vi "_PC_RTLoop_ReadVacuumSys.vi"(0 "string for turbo pump status":refnum<vi>, 1 "XYGraph for pressure":refnum<vi>[](array[refnum]), 2 "String refin":refnum<vi>, 3 "Function":enum16{"Init", "Get Data", "Close"}(ring), 5 "XYGraph for Turbo power":refnum<vi>, 9 "XYGraph for Turbo speed":refnum<vi>, 11 "error in (no error)":errorcluster) -> (15 "error out":errorcluster)   [LabVIEW 2018]
uses:
  <resource>/objmgr/ni.var.rc
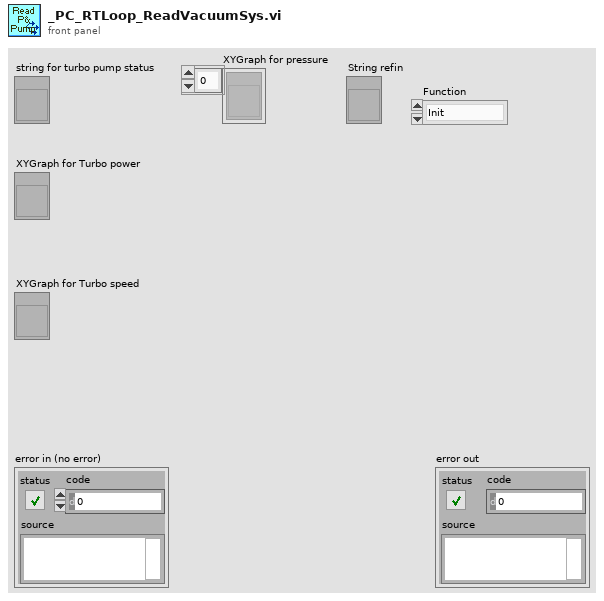
[diagram p1: front panel]
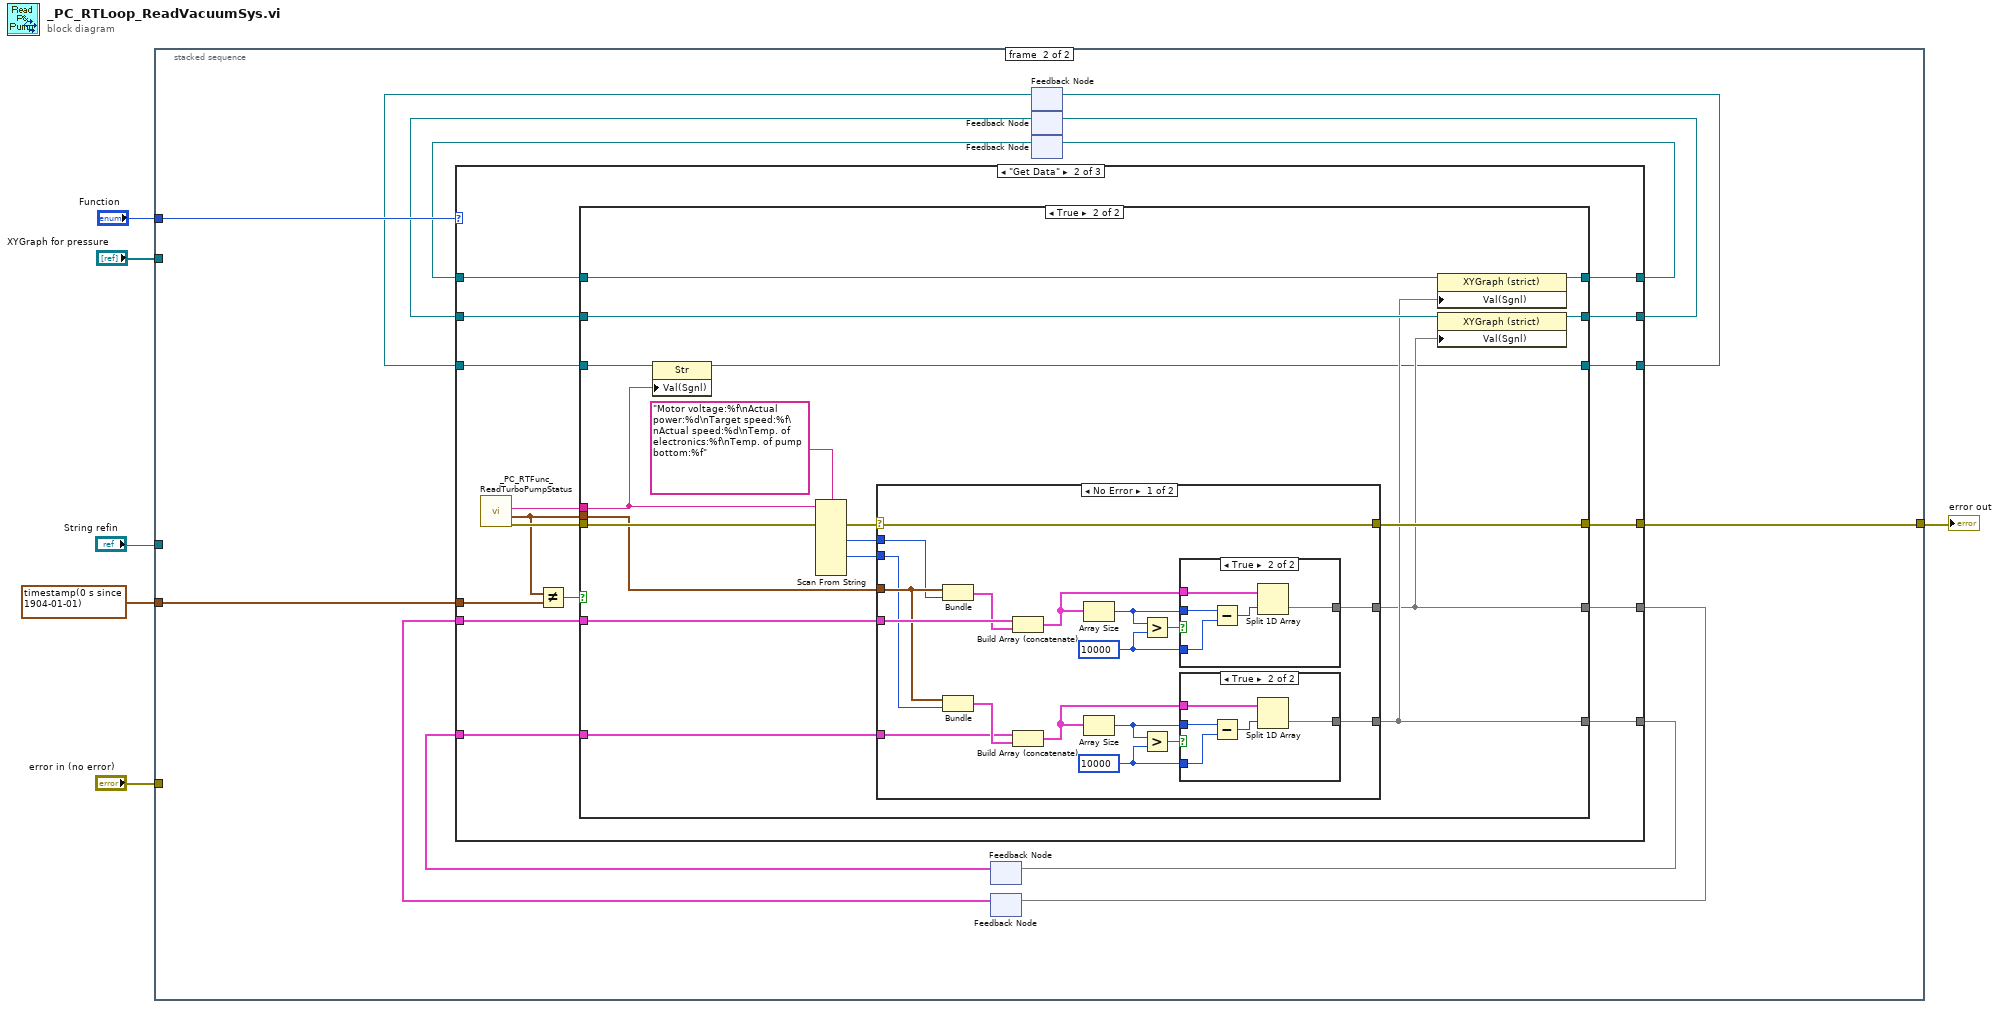
[diagram p0: block diagram]
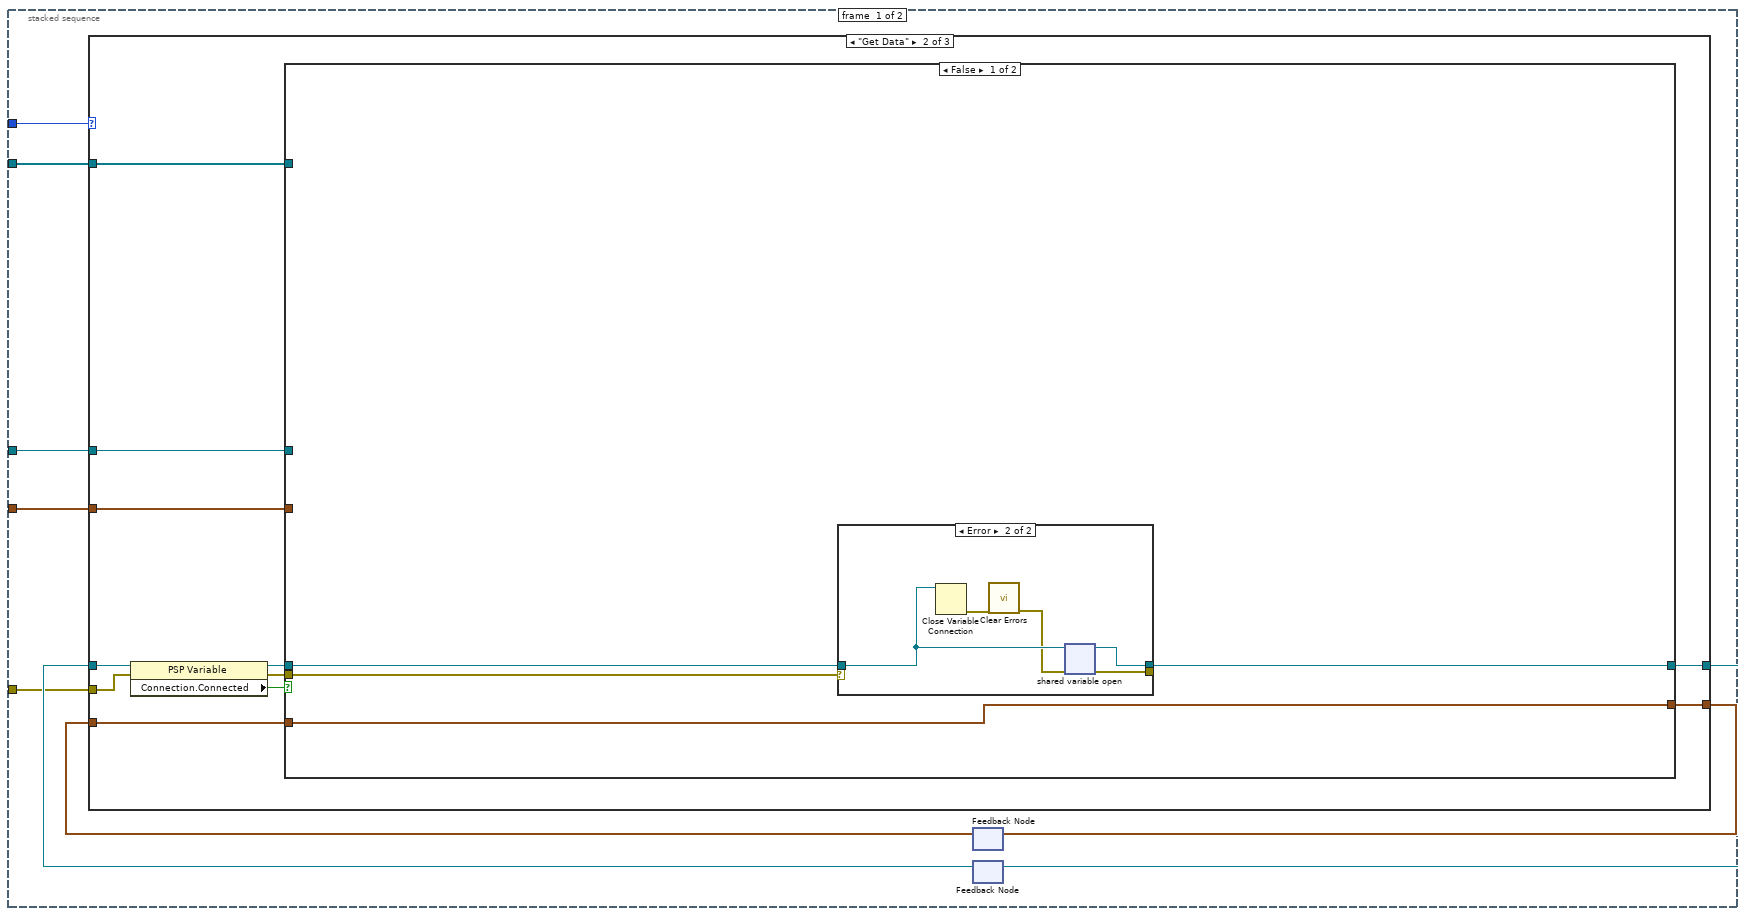
[diagram p2: hidden frame]
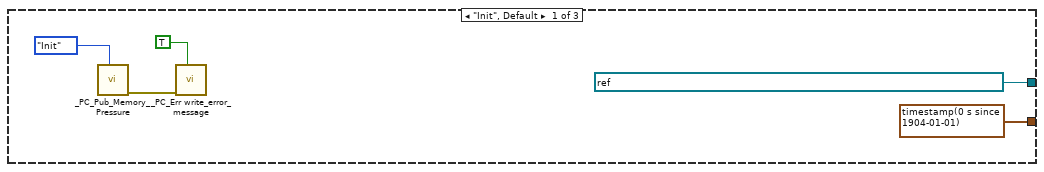
[diagram p3: hidden frame]
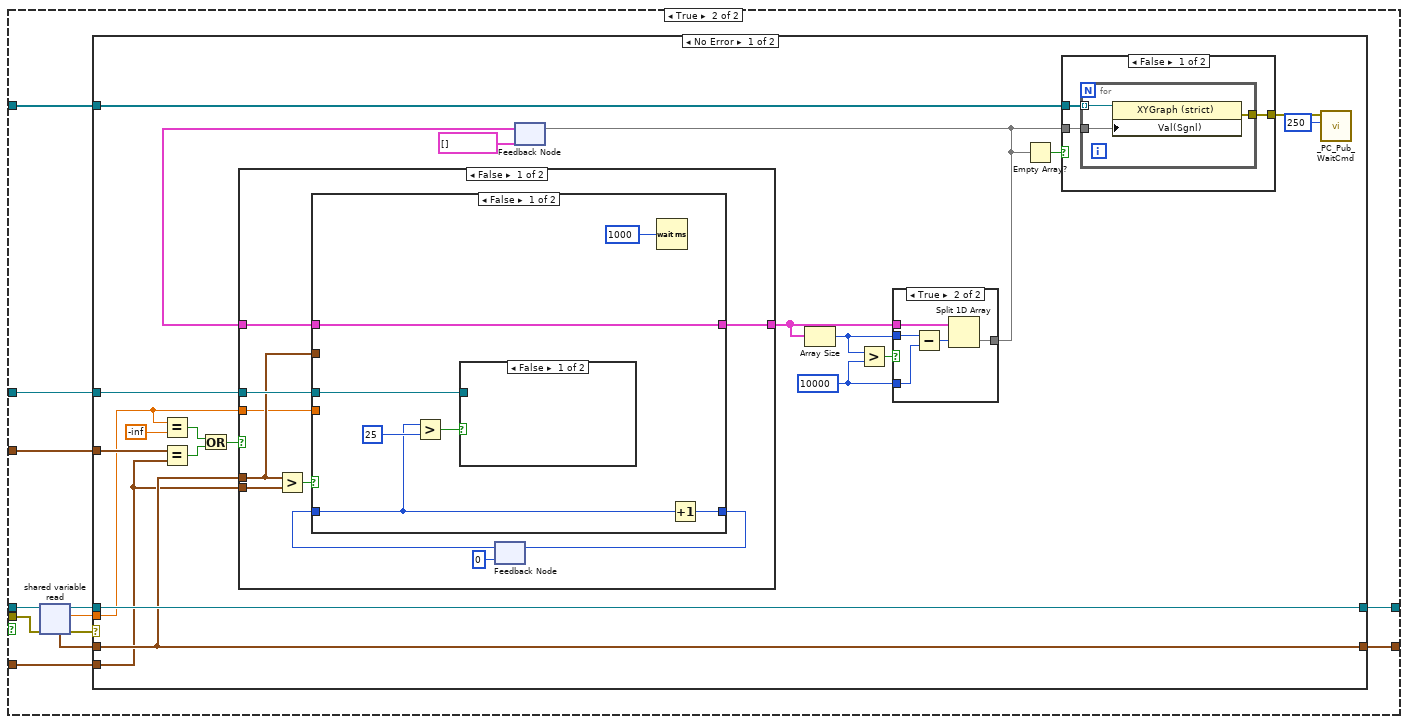
[diagram p5: hidden frame]
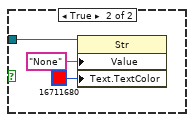
[diagram p8: hidden frame]
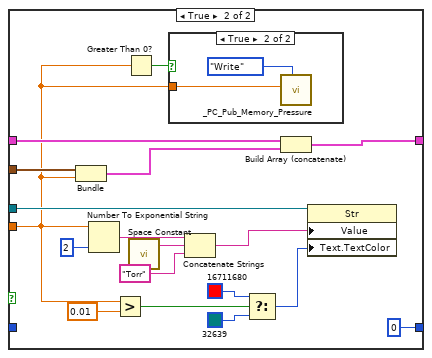
[diagram p9: hidden frame]
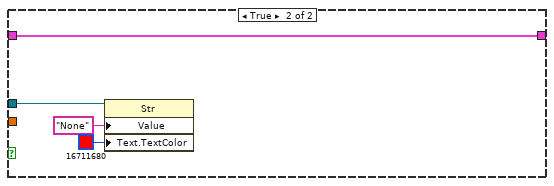
[diagram p11: hidden frame]
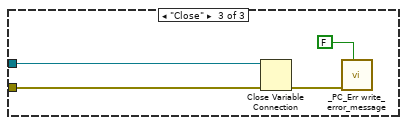
[diagram p13: hidden frame]
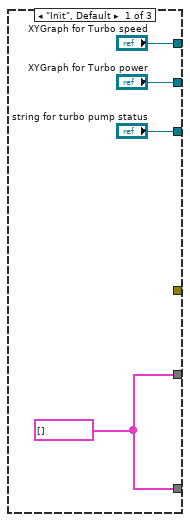
[diagram p14: hidden frame]
diagram:
  n1 = stacked-sequence {
    tunnel: "error in (no error)" -> [w13 _]
    tunnel: "Function" -> [w12 w149]
    tunnel: timestamp(0 s since 1904-01-01) -> [w9 w148]
    tunnel: "String refin" -> [w8 _]
    tunnel: "XYGraph for pressure" -> [w7 _]
    tunnel: [_ w143] -> w2
    frame #0 {
      n2 = feedback #1() -> (w10:timestamp)  [unwired: 1 in]
      n3 = feedback #2() -> (w14:refnum<k21>)  [unwired: 1 in]
      n4 = case shown="\"Get Data\"" w12 {
        tunnel: [refnum<k21> "ni.var.psp://NI-sbRIO/_RT_CtrlLoop_Pressure_Variables/Pressure_dbl" ("shared variable refnum in") w31 _] -> w15
        tunnel: w14 -> [_ w25 w136]
        tunnel: w13 -> [_ w23 w135]
        tunnel: [timestamp(0 s since 1904-01-01) w29 _] -> w11
        tunnel: w10 -> [_ w30 _]
        tunnel: w9 -> [_ w28 _]
        tunnel: w8 -> [_ w27 _]
        tunnel: w7 -> [_ w26 _]
        frame "Init", Default {
          n5 = call "_PC_Pub_Memory_Pressure.vi"("Function"=enum16{"Init", "Write", "Read"}."Init") -> ("error out"=w18:errorcluster)  [unwired: 9 in, 1 out]
          n6 = call "_PC_Err write_error_message.vi"("show msg( T )"=TRUE, "error in"=w18) -> ()  [unwired: 9 in, 1 out]
        }
        frame "Get Data" {
          n7 = property class="PSP Variable"(reference=w25, error in=w23) -> (reference out=w24:refnum<k21>, error out=w22:errorcluster, "Connection.Connected"=w21:bool)
          n8 = case shown="False" w21 {
            tunnel: [w32 w50] -> w31
            tunnel: w30 -> [w35 w48]
            tunnel: [w35 w47] -> w29
            tunnel: w28 -> [_ w46]
            tunnel: w27 -> [_ w45]
            tunnel: w26 -> [_ w44]
            tunnel: w24 -> [w33 w43]
            tunnel: w22 -> [w34 w42]
            frame False {
              n9 = case shown="Error" w34 {
                tunnel: w33 -> [w36 w40]
                tunnel: [w36 w38] -> w32
                tunnel: [_ w37] -> _
                frame No Error {
                }
                frame Error {
                  n10 = Close Variable Connection(11:w40) -> (0:w41:errorcluster)  [unwired: 1 in]
                  n11 = call <vilib>:"Clear Errors.vi"("error in (no error)"=w41) -> ("error out"=w39:errorcluster)  [unwired: 5 in, 1 out]
                  n12 = shared-variable-open(w40, w39) -> (w38:refnum<k21>, w37:errorcluster)
                }
              }
            }
            frame True {
              n13 = shared-variable-read(w43, w42) -> (w51:refnum<k21>, w52:errorcluster, w53:dbl, w49:timestamp)
              n14 = case shown="No Error" w52 {
                tunnel: w53 -> [w57 _]
                tunnel: w51 -> [w74 w131]
                tunnel: [w74 w131] -> w50
                tunnel: w49 -> [w72 w132]
                tunnel: w48 -> [w59 _]
                tunnel: [w72 w132] -> w47
                tunnel: w46 -> [w73 _]
                tunnel: w45 -> [w71 _]
                tunnel: w44 -> [w66 _]
                frame No Error {
                  w69 = 10000 ("y")
                  n15 = Equal?(x=w57, y=-inf) -> (x = y?=w56:bool)
                  n16 = Equal?(x=w73, y=w59) -> (x = y?=w55:bool)
                  n17 = Or(x=w56, y=w55) -> (x .or. y?=w54:bool)
                  n18 = feedback #3(cluster{timestamp, "Double":dbl}[] []) -> (w62:cluster{timestamp, "Double":dbl}[])
                  n19 = case shown="False" w54 {
                    tunnel: w72 -> [w91 _]
                    tunnel: w71 -> [w92 w128]
                    tunnel: w57 -> [w90 _]
                    tunnel: [w89 w127] -> w67
                    tunnel: w62 -> [w88 w127]
                    tunnel: w59 -> [w87 _]
                    frame False {
                      n20 = Greater?(x=w91, y=w87) -> (0:w96:bool)
                      n21 = feedback #4(0) -> (w94:i32)
                      n22 = case shown="False" w96 {
                        tunnel: w91 -> [_ w124]
                        tunnel: w90 -> [_ w113]
                        tunnel: [w103 w122] -> w89
                        tunnel: w88 -> [w103 w121]
                        tunnel: w92 -> [w102 w120]
                        tunnel: [w100 0] -> w95
                        tunnel: w94 -> [w98 _]
                        frame False {
                          n23 = Greater?(x=w98, y=25 ("x")) -> (0:w97:bool)
                          n24 = case shown="False" w97 {
                            tunnel: w102 -> [_ w104]
                            frame False {
                            }
                            frame True {
                              n25 = property class="Str"(reference=w104, "Value"="None", "Text.TextColor"=u32 16711680) -> ()  [unwired: 1 in, 2 out]
                            }
                          }
                          n26 = Wait (ms)(milliseconds to wait=u32 1000) -> ()  [unwired: 1 out]
                          n27 = Increment(x=w98) -> (x+1=w100:i32)
                        }
                        frame True {
                          n28 = Bundle(w124, "Double"=w113) -> (w123:cluster{timestamp, "Double":dbl})  [unwired: 1 in]
                          n29 = Number To Exponential String(number=w113, precision (6)=i16 2) -> (E-format string=w115:string)  [unwired: 2 in]
                          n30 = Greater?(x=w113, y=0.01) -> (0:w111:bool)
                          n31 = Greater Than 0?(x=w113) -> (x > 0?=w119:bool)
                          n32 = call <vilib>:"Space Constant.vi"() -> ("String"=w116:string)
                          n33 = case shown="True" w119 {
                            tunnel: w113 -> [_ w125]
                            frame False {
                            }
                            frame True {
                              n34 = call "_PC_Pub_Memory_Pressure.vi"("Function"=enum16{"Init", "Write", "Read"}."Write", "Pressure in"=w125) -> ()  [unwired: 8 in, 2 out]
                            }
                          }
                          n35 = Concatenate Strings(w115, w116, "Torr" ("string")) -> (w114:string)
                          n36 = Select(t=u32 16711680, s=w111, f=u32 32639) -> (s? t:f=w108:u32)
                          n37 = Build Array (concatenate)(w121, w123) -> (w122:cluster{timestamp, "Double":dbl}[])
                          n38 = property class="Str"(reference=w120, "Value"=w114, "Text.TextColor"=w108) -> ()  [unwired: 1 in, 2 out]
                        }
                      }
                      n39 = feedback-in #4(w95) -> ()
                    }
                    frame True {
                      n40 = property class="Str"(reference=w128, "Value"="None", "Text.TextColor"=u32 16711680) -> ()  [unwired: 1 in, 2 out]
                    }
                  }
                  n41 = Array Size(array=w67) -> (size(s)=w68:i32)
                  n42 = Greater?(x=w68, y=w69) -> (0:w70:bool)
                  n43 = case shown="True" w70 {
                    tunnel: w67 -> [w81 w86]
                    tunnel: w69 -> [_ w85]
                    tunnel: w68 -> [_ w84]
                    tunnel: [w81 w82] -> w63
                    frame False {
                    }
                    frame True {
                      n44 = Subtract(x=w84, y=w85) -> (x-y=w83:i32)
                      n45 = Split 1D Array(array=w86, index=w83) -> (second subarray=w82:cluster{timestamp, "Double":dbl}[])  [unwired: 1 out]
                    }
                  }
                  n46 = feedback-in #3(w63) -> ()
                  n47 = Empty Array?(array=w63) -> (empty?=w65:bool)
                  n48 = case shown="False" w65 {
                    tunnel: w66 -> [w77 _]
                    tunnel: w63 -> [w76 _]
                    tunnel: [w75 _] -> w61
                    frame False {
                      n49 = for {
                        tunnel: w77 -> [w80] mode=indexing
                        tunnel: w76 -> [w79]
                        tunnel: [w78] -> w75
                        n50 = property class="XYGraph (strict)"(reference=w80, "Val(Sgnl)"=w79) -> (error out=w78:errorcluster)  [unwired: 1 in, 1 out]
                      }
                    }
                    frame True {
                    }
                  }
                  n51 = call "_PC_Pub_WaitCmd.vi"("milliseconds to wait"=u32 250, "error in (no error)"=w61) -> ()  [unwired: 9 in, 1 out]
                }
                frame Error {
                }
              }
            }
          }
        }
        frame "Close" {
          n52 = Close Variable Connection(8:w135, 11:w136) -> (0:w134:errorcluster)
          n53 = call "_PC_Err write_error_message.vi"("show msg( T )"=FALSE, "error in"=w134) -> ()  [unwired: 9 in, 1 out]
        }
      }
      n54 = feedback-in #1(w11) -> ()
      n55 = feedback-in #2(w15) -> ()
    }
    frame #1 {
      n56 = feedback #5() -> (w145:cluster{"Time Stamp":timestamp, i32}[])  [unwired: 1 in]
      n57 = feedback #6() -> (w144:cluster{"Time Stamp":timestamp, i32}[])  [unwired: 1 in]
      n58 = feedback #7() -> (w137:refnum<vi>)  [unwired: 1 in]
      n59 = feedback #8() -> (w139:refnum<vi>)  [unwired: 1 in]
      n60 = feedback #9() -> (w141:refnum<vi>)  [unwired: 1 in]
      n61 = case shown="\"Get Data\"" w149 {
        tunnel: w148 -> [_ w162 _]
        tunnel: w144 -> [_ w167 _]
        tunnel: w145 -> [_ w166 _]
        tunnel: [w153 w165 _] -> w146
        tunnel: [w153 w164 _] -> w147
        tunnel: [_ w163 _] -> w143
        tunnel: ["XYGraph for Turbo speed" w159 _] -> w142
        tunnel: ["XYGraph for Turbo power" w158 _] -> w140
        tunnel: ["string for turbo pump status" w157 _] -> w138
        tunnel: w141 -> [_ w156 _]
        tunnel: w139 -> [_ w155 _]
        tunnel: w137 -> [_ w154 _]
        frame "Init", Default {
          w153 = cluster{"Time Stamp":timestamp, i32}[] []
        }
        frame "Get Data" {
          n62 = call "_PC_RTFunc_ReadTurboPumpStatus.vi"() -> ("error out"=w168:errorcluster, "Time Stamp"=w160:timestamp, "TurboStatus_string"=w169:string)  [unwired: 8 in, 1 out]
          n63 = Not Equal?(x=w160, y=w162) -> (x != y?=w161:bool)
          n64 = case shown="True" w161 {
            tunnel: w169 -> [_ w187]
            tunnel: w168 -> [w173 w192]
            tunnel: w154 -> [w170 w188]
            tunnel: w155 -> [w171 w185]
            tunnel: w156 -> [w172 w184]
            tunnel: w160 -> [_ w186]
            tunnel: w167 -> [w175 w183]
            tunnel: w166 -> [w174 w182]
            tunnel: [w175 w179] -> w165
            tunnel: [w174 w180] -> w164
            tunnel: [w173 w181] -> w163
            tunnel: [w172 w178] -> w159
            tunnel: [w171 w177] -> w158
            tunnel: [w170 w176] -> w157
            frame False {
            }
            frame True {
              n65 = property class="Str"(reference=w188, "Val(Sgnl)"=w187) -> (reference out=w176:refnum<vi>)  [unwired: 1 in, 1 out]
              n66 = Scan From String(format string="Motor voltage:%f\nActual power:%d\nTarget speed:%f\nActual speed:%d\nTemp. of electronics:%f\nTemp. of pump bottom:%f", input string=w187, error in=w192) -> (error out=w191:errorcluster, output 2=w190:i32, output 4=w189:i32)  [unwired: 11 in, 2 out]
              n67 = case shown="No Error" w191 {
                selector: w191 -> [w194 w224]
                tunnel: w183 -> [w211 w226]
                tunnel: w182 -> [w195 w225]
                tunnel: w186 -> [w209 _]
                tunnel: [w197 w225] -> w180
                tunnel: w190 -> [w208 _]
                tunnel: w189 -> [w207 _]
                tunnel: [w202 w226] -> w179
                tunnel: [w194 w224] -> w181
                frame No Error {
                  w200 = 10000 ("y")
                  w205 = 10000 ("y")
                  n68 = Bundle("Time Stamp"=w209, w208) -> (w210:cluster{"Time Stamp":timestamp, i32})  [unwired: 1 in]
                  n69 = Bundle("Time Stamp"=w209, w207) -> (w196:cluster{"Time Stamp":timestamp, i32})  [unwired: 1 in]
                  n70 = Build Array (concatenate)(w211, w210) -> (w203:cluster{"Time Stamp":timestamp, i32}[])
                  n71 = Build Array (concatenate)(w195, w196) -> (w198:cluster{"Time Stamp":timestamp, i32}[])
                  n72 = Array Size(array=w203) -> (size(s)=w204:i32)
                  n73 = Array Size(array=w198) -> (size(s)=w199:i32)
                  n74 = Greater?(x=w204, y=w205) -> (0:w206:bool)
                  n75 = Greater?(x=w199, y=w200) -> (0:w201:bool)
                  n76 = case shown="True" w206 {
                    tunnel: w205 -> [_ w223]
                    tunnel: w204 -> [_ w222]
                    tunnel: [w218 w220] -> w202
                    tunnel: w203 -> [w218 w219]
                    frame False {
                    }
                    frame True {
                      n77 = Subtract(x=w222, y=w223) -> (x-y=w221:i32)
                      n78 = Split 1D Array(array=w219, index=w221) -> (second subarray=w220:cluster{"Time Stamp":timestamp, i32}[])  [unwired: 1 out]
                    }
                  }
                  n79 = case shown="True" w201 {
                    tunnel: w200 -> [_ w217]
                    tunnel: w199 -> [_ w216]
                    tunnel: [w212 w214] -> w197
                    tunnel: w198 -> [w212 w213]
                    frame False {
                    }
                    frame True {
                      n80 = Subtract(x=w216, y=w217) -> (x-y=w215:i32)
                      n81 = Split 1D Array(array=w213, index=w215) -> (second subarray=w214:cluster{"Time Stamp":timestamp, i32}[])  [unwired: 1 out]
                    }
                  }
                }
                frame Error {
                }
              }
              n82 = property class="XYGraph (strict)"(reference=w184, "Val(Sgnl)"=w180) -> (reference out=w178:refnum<vi>)  [unwired: 1 in, 1 out]
              n83 = property class="XYGraph (strict)"(reference=w185, "Val(Sgnl)"=w179) -> (reference out=w177:refnum<vi>)  [unwired: 1 in, 1 out]
            }
          }
        }
        frame "Close" {
        }
      }
      n84 = feedback-in #5(w147) -> ()
      n85 = feedback-in #6(w146) -> ()
      n86 = feedback-in #7(w138) -> ()
      n87 = feedback-in #8(w140) -> ()
      n88 = feedback-in #9(w142) -> ()
    }
  }
  "error out" <- w2
